vi "Calculate Curvature.vi"(10 "Odometry":T1, 11 "Target Point":T2) -> (2 "Curvature":dbl, 3 "Lookahead Point Robot Frame":cluster{"x out":dbl, "y out":dbl})   [LabVIEW 2019, in "Pure Pursuit.lvlib"]
uses:
  Pure Pursuit.lvlib
  Typedef/Path Point.ctl
  Odometry/Typedef/Odometry.ctl
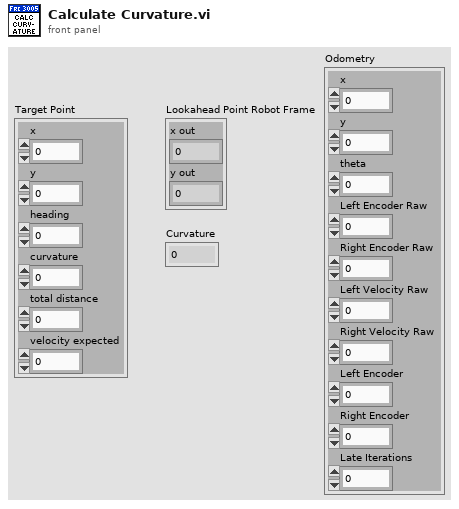
[diagram p1: front panel]
types:
  T1 = typedef "Odometry.ctl" = cluster{"x":dbl, "y":dbl, "theta":dbl, "Left Encoder Raw":i32, "Right Encoder Raw":i32, "Left Velocity Raw":i32, "Right Velocity Raw":i32, "Left Encoder":dbl, "Right Encoder":dbl, "Late Iterations":i16}
  T2 = typedef "Pure Pursuit.lvlib/Path Point.ctl" = cluster{"x":dbl, "y":dbl, "heading":dbl, "curvature":dbl, "total distance":dbl, "velocity expected":dbl}
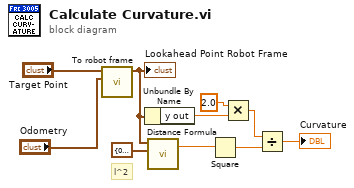
[diagram p0: block diagram]
diagram:
  # "l^2"
  n1 = call "To robot frame.vi"("Odometry"="Odometry", "Lookahead Point"="Target Point") -> ("Lookahead Point Out"=w6:cluster{"x out":dbl, "y out":dbl})  [unwired: 9 in]
  "Lookahead Point Robot Frame" <- w6
  n2 = Unbundle By Name(w6) -> ("y out"=w8:dbl)
  n3 = call "Distance Formula.vi"("Point2"=cluster{"x":dbl, "y":dbl} {"x"=0.0, "y"=0.0}, "Point1"=w6) -> ("Distance"=w2:dbl)  [unwired: 3 in]
  n4 = Square(x=w2) -> (x^2=w5:dbl)
  n5 = Multiply(x=2.0, y=w8) -> (x*y=w4:dbl)
  n6 = Divide(x=w4, y=w5) -> (x/y=→"Curvature":dbl)
